vi "Insert NaN.vi"(1 "array in":dbl[](array[numeric])) -> (0 "array out":dbl[](array[numeric]))   [LabVIEW 2015]
panel:
  # "Inserts NaN into an array"
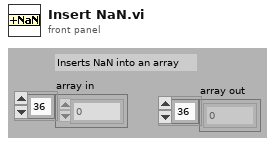
[diagram p1: front panel]
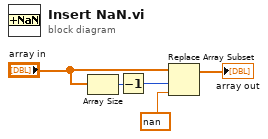
[diagram p0: block diagram]
diagram:
  n1 = Array Size(array="array in") -> (size(s)=w2:i32)
  n2 = Decrement(x=w2) -> (x-1=w1:i32)
  n3 = Replace Array Subset(array="array in", new element=nan, index=w1) -> (→"array out":dbl[])
